vi "UnixUTCToLVTime.vi"(8 "error in (no error)":errorcluster, 11 "Unix Time (in milliseconds)":u64) -> (0 "error out":errorcluster, 3 "Local Timestamp":timestamp)   [LabVIEW 2013, in "BSON.lvlib" / "tBSONTimestamp.lvclass"]
uses:
  tBSONTimestamp.lvclass
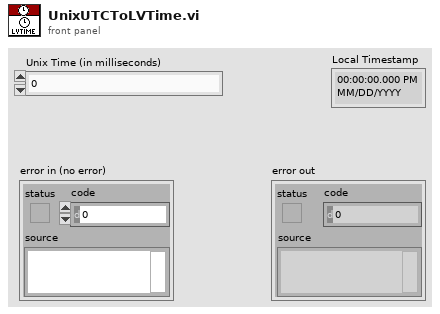
[diagram p1: front panel]
types:
  T1 = typedef "LVDateTimeRec.ctl" = cluster{"fractional second":dbl, "second":i32, "minute":i32, "hour":i32, "day of month":i32, "month":i32, "year":i32, "day of week":i32, "day of year":i32, "DST":i32}
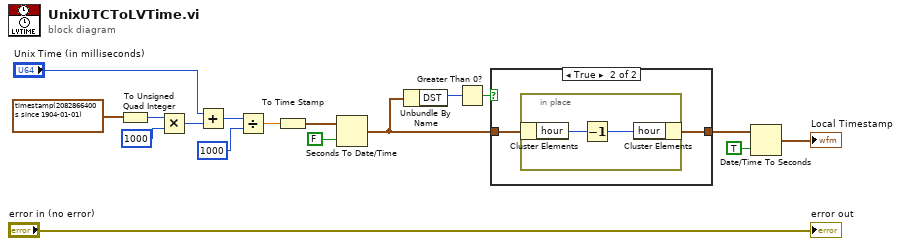
[diagram p0: block diagram]
diagram:
  n1 = To Unsigned Quad Integer(1:timestamp(2082866400 s since 1904-01-01) ("time stamp")) -> (0:w16:u64)
  n2 = Multiply(x=w16, y=u64 1000) -> (x*y=w14:u64)
  n3 = Add(x="Unix Time (in milliseconds)", y=w14) -> (x+y=w12:u64)
  n4 = Divide(x=w12, y=u64 1000) -> (x/y=w10:dbl)
  n5 = To Time Stamp(1:w10) -> (0:w9:timestamp)
  n6 = Seconds To Date/Time(time stamp (now)=w9, to UTC (F)=FALSE) -> (date time rec=w2:T1)
  n7 = Unbundle By Name(w2) -> ("DST"=w4:i32)
  n8 = Greater Than 0?(x=w4) -> (x > 0?=w3:bool)
  n9 = case shown="True" w3 {
    tunnel: w2 -> [w18 w20]
    tunnel: [w18 w19] -> w1
    frame False {
    }
    frame True {
      n10 = in-place {
        n11 = in-place-cluster #1(w20) -> ("hour"=w22:i32)
        n12 = Decrement(x=w22) -> (x-1=w21:i32)
        n13 = in-place-cluster #1("hour"=w21) -> (w19:T1)
      }
    }
  }
  n14 = Date/Time To Seconds(1:TRUE ("is UTC (F)"), 2:w1) -> (0:→"Local Timestamp":timestamp)
  "error out" <- "error in (no error)"
